vi "CreateConfocal.vi"(8 "error in (no error)":errorcluster, 11 "CurrentImage":dbl[](array[numeric])) -> (0 "error out":errorcluster, 3 "imageout":dbl[][](array[numeric]))   [LabVIEW 2011]
uses:
  Variables/ccdChipPixels.vi
  Variables/AxisSteps.vi
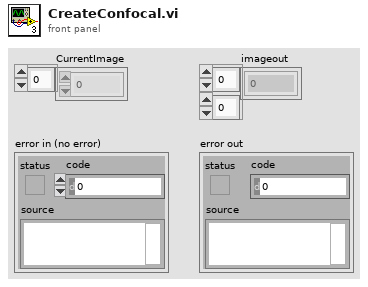
[diagram p1: front panel]
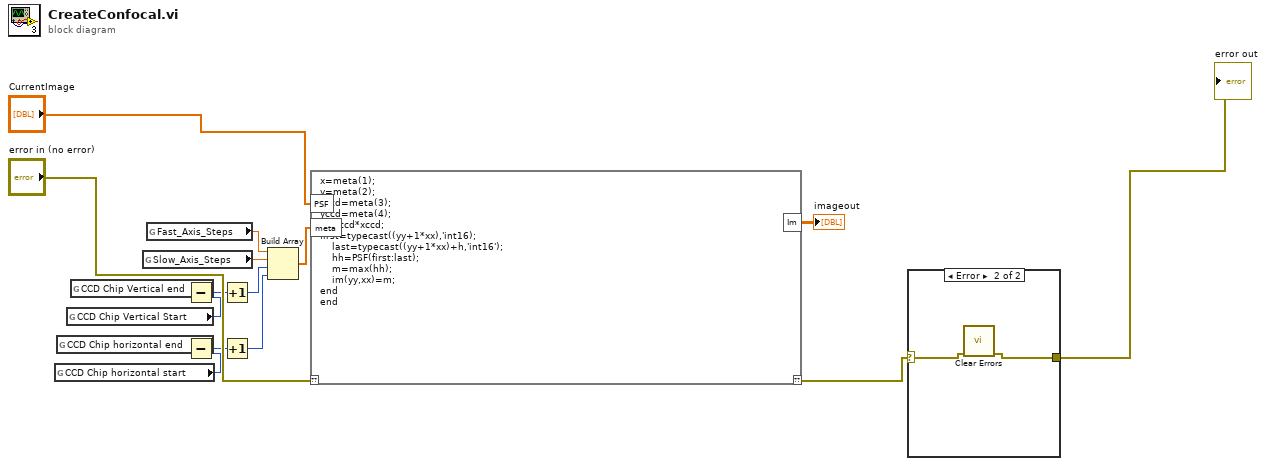
[diagram p0: block diagram]
diagram:
  n1 = global read "ccdChipPixels.vi" "CCD Chip horizontal start"() -> (w2:i32)
  n2 = global read "ccdChipPixels.vi" "CCD Chip horizontal end"() -> (w3:i32)
  n3 = global read "ccdChipPixels.vi" "CCD Chip Vertical Start"() -> (w5:i32)
  n4 = global read "ccdChipPixels.vi" "CCD Chip Vertical end"() -> (w6:i32)
  n5 = global read "AxisSteps.vi" "Slow_Axis_Steps"() -> (w8:dbl)
  n6 = global read "AxisSteps.vi" "Fast_Axis_Steps"() -> (w7:dbl)
  n7 = Subtract(x=w6, y=w5) -> (x-y=w10:i32)
  n8 = Subtract(x=w3, y=w2) -> (x-y=w11:i32)
  n9 = Increment(x=w10) -> (x+1=w4:i32)
  n10 = Increment(x=w11) -> (x+1=w1:i32)
  n11 = Build Array(w7, w8, w4, w1) -> (w9:dbl[])
  n12 = script code="x=meta(1);\ny=meta(2);\nxccd=meta(3);\nyccd=meta(4);\nh=yccd*xccd;\nfirst=typecast((yy+1*xx),'int16);\n    last=typecast((yy+1*xx)+h,'int16');\n    hh=PSF(first:last);\n    m=max(hh);\n    im(yy,xx)=m;\nend\nend"("??"="error in (no error)", "PSF"="CurrentImage", "meta"=w9) -> ("??"=w13:errorcluster, "Im"=→"imageout":dbl[][])
  n13 = case shown="Error" w13 {
    selector: w13 -> [w17 w19]
    tunnel: [w17 w18] -> w14
    frame No Error {
    }
    frame Error {
      n14 = call <vilib>:"Clear Errors.vi"("error in (no error)"=w19) -> ("error out"=w18:errorcluster)  [unwired: 6 in]
    }
  }
  "error out" <- w14
